vi "svx_DAQ_SetUnits.vi"(4 "Channel Information In":T1={"Initialized?"=FALSE, "DAQmx Channel"="", "Channel Type"=0, "Max"=5.0, "Sensitivity"=1000.0, "Excitation"=FALSE, "Coupling"=enum."DC", "Location"="", "Orientation"="", "excitation"=enum."Off"} {"Max" min=0.0 format="± %^#_4g"; "Channel Type" items=["Voltage (V)"=0, "Charge (C)"=9, "-"=99, "SPL (Pa)"=3, "Force (lbf)"=6, "Force (N)"=1, "Acceleration (g) - IEPE"=2, "Acceleration (g) - Charge"=12, "Acceleration (g) - 4 wire DC Voltage"=22, "Velocity (in/s)"=7, "Velocity (mm/s)"=8, "Prox Probe (mil)"=4, "Prox Probe (mm)"=5]}) -> (1 "Channel Information Out":T1={"Initialized?"=FALSE, "DAQmx Channel"="", "Channel Type"=0, "Max"=5.0, "Sensitivity"=1000.0, "Excitation"=FALSE, "Coupling"=enum."DC", "Location"="", "Orientation"="", "excitation"=enum."Off"} {"Max" min=0.0 format="± %^#_4g"; "Channel Type" items=["Voltage (V)"=0, "Charge (C)"=9, "-"=99, "SPL (Pa)"=3, "Force (lbf)"=6, "Force (N)"=1, "Acceleration (g) - IEPE"=2, "Acceleration (g) - Charge"=12, "Acceleration (g) - 4 wire DC Voltage"=22, "Velocity (in/s)"=7, "Velocity (mm/s)"=8, "Prox Probe (mil)"=4, "Prox Probe (mm)"=5]})   [LabVIEW 2017, in "SVX NI-DAQmx AI Configuration XControl.xctl"]
uses:
  <vilib>/addons/Sound and Vibration/svt_DAQmx/Configuration XControl/SVX NI-DAQmx AI Configuration XControl.xctl
  <vilib>/addons/Sound and Vibration/svt_DAQmx/Configuration XControl/Controls/svx_DAQ_ChannelInfo.ctl
  <vilib>/addons/Sound and Vibration/svt_DAQmx/Configuration XControl/Controls/svx_DAQ_ChannelType.ctl
  <vilib>/addons/Sound and Vibration/svt_DAQmx/Configuration XControl/Controls/svx_DAQ_Coupling.ctl
  <vilib>/addons/Sound and Vibration/svt_DAQmx/Configuration XControl/Controls/svx_DAQ_Excitation.ctl
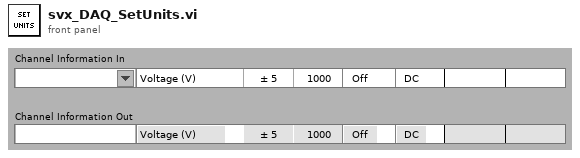
[diagram p1: front panel]
types:
  T1 = typedef "SVX NI-DAQmx AI Configuration XControl.xctl/svx_DAQ_ChannelInfo.ctl" = cluster{"Initialized?":bool, "DAQmx Channel":tag, "Channel Type":T2, "Max":dbl, "Sensitivity":dbl, "Excitation":bool, "Coupling":T3, "Location":string, "Orientation":string, "excitation":T4}
  T2 = typedef "SVX NI-DAQmx AI Configuration XControl.xctl/svx_DAQ_ChannelType.ctl" = u16
  T3 = typedef "SVX NI-DAQmx AI Configuration XControl.xctl/svx_DAQ_Coupling.ctl" = enum16{"AC", "DC"}
  T4 = typedef "svx_DAQ_Excitation.ctl" = enum16{"Off", "Min", "Max"}
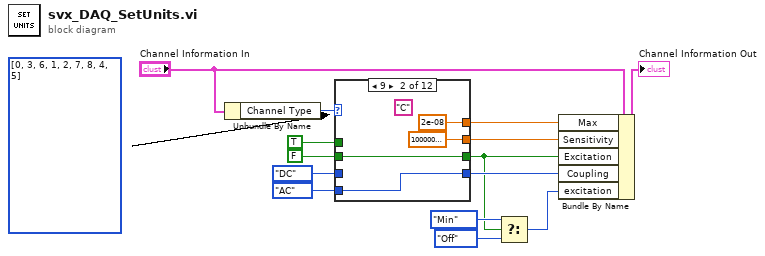
[diagram p0: block diagram]
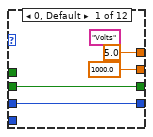
[diagram p2: hidden frame]
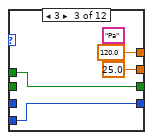
[diagram p3: hidden frame]
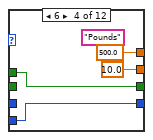
[diagram p4: hidden frame]
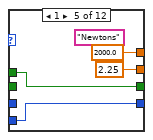
[diagram p5: hidden frame]
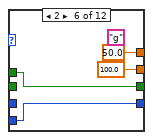
[diagram p6: hidden frame]
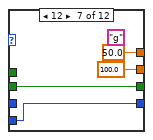
[diagram p7: hidden frame]
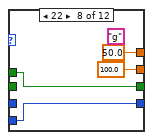
[diagram p8: hidden frame]
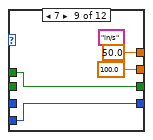
[diagram p9: hidden frame]
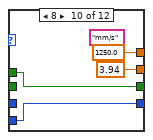
[diagram p10: hidden frame]
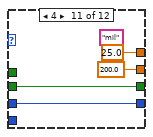
[diagram p11: hidden frame]
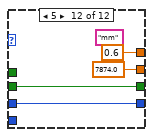
[diagram p12: hidden frame]
diagram:
  (unwired) T2[] [0, 3, 6, 1, 2, 7, 8, 4, 5] items=["Voltage (V)"=0, "SPL (Pa)"=3, "Force (lbf)"=6, "Force (N)"=1, "Acceleration (g)"=2, "Velocity (in/s)"=7, "Velocity (mm/s)"=8, "Prox Probe (mil)"=4, "Prox Probe (mm)"=5]
  n1 = Unbundle By Name("Channel Information In") -> ("Channel Type"=w13:T2)
  n2 = case shown="9" w13 {
    tunnel: [5.0 ("Max") 2e-08 ("Max") 120.0 ("Max") 500.0 ("Max") 2000.0 ("Max") 50.0 ("Max") 50.0 ("Max") 50.0 ("Max") 50.0 ("Max") 1250.0 ("Max") 25.0 ("Max") 0.6 ("Max")] -> w14
    tunnel: [1000.0 ("Sensitivity") 1000000000000.0 ("Sensitivity") 25.0 ("Sensitivity") 10.0 ("Sensitivity") 2.25 ("Sensitivity") 100.0 ("Sensitivity") 100.0 ("Sensitivity") 100.0 ("Sensitivity") 100.0 ("Sensitivity") 3.94 ("Sensitivity") 200.0 ("Sensitivity") 7874.0 ("Sensitivity")] -> w12
    tunnel: FALSE ("IEPE") -> [w16 w20 _ _ _ _ w39 _ _ _ w56 w60]
    tunnel: [w16 w20 w24 w28 w32 w36 w39 w43 w48 w52 w56 w60] -> w1
    tunnel: svx_DAQ_Coupling."DC" ("Coupling") -> [w15 _ _ _ _ _ _ _ _ _ w55 w59]
    tunnel: [w15 w19 w23 w27 w31 w35 w40 w44 w47 w51 w55 w59] -> w9
    tunnel: TRUE ("IEPE") -> [_ _ w24 w28 w32 w36 _ w43 w48 w52 _ _]
    tunnel: svx_DAQ_Coupling."AC" ("Coupling") -> [_ w19 w23 w27 w31 w35 w40 w44 w47 w51 _ _]
    frame 0, Default {
      (unwired) "Volts"
    }
    frame 9 {
      (unwired) "C"
    }
    frame 3 {
      (unwired) "Pa"
    }
    frame 6 {
      (unwired) "Pounds"
    }
    frame 1 {
      (unwired) "Newtons"
    }
    frame 2 {
      (unwired) "g"
    }
    frame 12 {
      (unwired) "g"
    }
    frame 22 {
      (unwired) "g"
    }
    frame 7 {
      (unwired) "in/s"
    }
    frame 8 {
      (unwired) "mm/s"
    }
    frame 4 {
      (unwired) "mil"
    }
    frame 5 {
      (unwired) "mm"
    }
  }
  n3 = Select(t=svx_DAQ_Excitation."Min" ("excitation"), s=w1, f=svx_DAQ_Excitation."Off" ("excitation")) -> (s? t:f=w2:T4)
  n4 = Bundle By Name(cluster="Channel Information In", "Max"=w14, "Sensitivity"=w12, "Excitation"=w1, "Coupling"=w9, "excitation"=w2) -> (→"Channel Information Out":T1)
